vi "SLL DE AI Moving Average V3.0.vi"(8 "error in (no error)":errorcluster, 11 "Input Array":dbl[][](array[numeric])) -> (0 "error out":errorcluster, 3 "Averaged Array":dbl[][](array[numeric]))   [LabVIEW 2013]
uses:
  Controls/SLL DE DAQ Parameters LV2Global Options.ctl
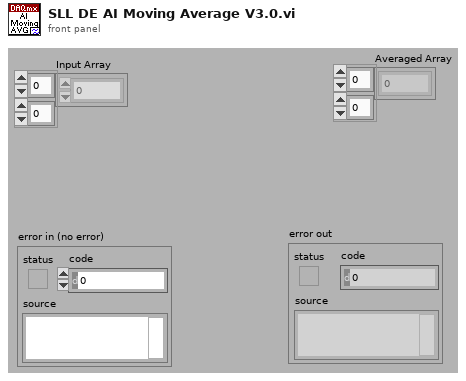
[diagram p1: front panel]
types:
  T1 = typedef "SLL DE DAQ Parameters LV2Global Options.ctl" = enum16{"Read", "Write"}
  T2 = typedef "SLL DE DAQ Engine Parameters.ctl" = cluster{"Enable Engines":cluster{"AI Enable":bool, "AO Enable":bool, "DI Enable":bool, "DO Enable":bool}, "DAQ Control Type":cluster{"Analog Input":enum16{"Finite", "Continuous", "Driver"}, "Analog Output":enum16{"Finite", "Continuous", "Driver"}, "Digital Input":enum16{"Finite", "Continuous", "Driver"}, "Digital Output":enum16{"Finite", "Continuous", "Driver"}}, "DAQ Parameters":cluster{"AI Sampling Rate (Samples/Sec)":dbl, "MvgAVG Window Size (# of Points)":i32, "Enable Filter":bool, "Enable MvgAVG":bool, "Circular Buffer Size (Sec)":dbl, "AO Sampling Rate (Samples/Sec)":dbl, "Graph Update Rate (Samples/Sec)":dbl, "File Logging Rate (Samples/Sec)":i32}, "AO Safe Values":cluster{"Analog Outputs Name":T3, "Analog Outputs Safe Value":dbl}[], "DO Safe Values":cluster{"Digital Outputs Name":T4, "Digital Outputs Safe Value":bool}[], "DO Interconnected Lines":cluster{"First DO Line":string, "Second DO Line":string}[], "AI Channels Unit":cluster{"Channel Name":T5, "Channel Type":T6}[], "Units Information":cluster{"Channel Type":T6, "Unit Text":string, "Maximum":dbl, "Minmum":dbl, "Increments":dbl}[]}
  T3 = typedef "SLL DE List of Analog Outputs.ctl" = enum16{"None"}
  T4 = typedef "SLL DE List of Digital Outputs.ctl" = enum16{"STATION1_START TEST", "STATION1_STOP TEST", "STATION1_LIGHT1", "STATION1_LIGHT2", "STATION1_LIGHT3", "STATION1_SELECT_TEST", "STATION2_START TEST", "STATION2_STOP TEST", "STATION2_LIGHT1", "STATION2_LIGHT2", "STATION2_LIGHT3", "STATION2_SELECT_TEST", "STATION3_START TEST", "STATION3_STOP TEST", "STATION3_LIGHT1", "STATION3_LIGHT2", "STATION3_LIGHT3", "STATION3_SELECT_TEST", "STATION4_START TEST", "STATION4_STOP TEST", "STATION4_LIGHT1", "STATION4_LIGHT2", "STATION4_LIGHT3", "STATION4_SELECT_TEST"}
  T5 = typedef "SLL DE List of Analog Inputs.ctl" = enum16{"None"}
  T6 = typedef "SLL DE List of AI Channel Type.ctl" = enum16{"Pressure", "Flow", "Temperature", "Time Scale", "Voltage", "Current", "Frequency", "Sound", "Speed", "Torque", "Distance", "Channel Type 1", "Channel Type 2", "Channel Type 3"}
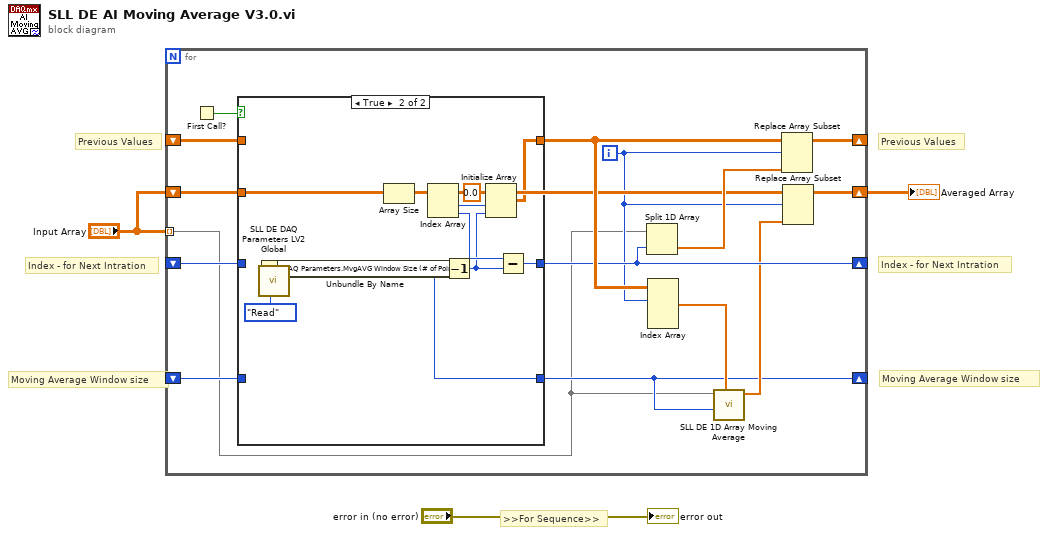
[diagram p0: block diagram]
diagram:
  # ">>For Sequence>>"
  # "Index - for Next Intration"
  # "Index - for Next Intration"
  # "Previous Values"
  # "Previous Values"
  # "Moving Average Window size"
  # "Moving Average Window size"
  n1 = for {
    tunnel: "Input Array" -> [w4] mode=indexing
    shift-right: [w15] -> _
    shift-left: _ -> [w17]
    shift-right: [w12] -> _
    shift-left: _ -> [w11]
    shift-right: [w5] -> _
    shift-left: _ -> [w6]
    shift-right: [w7] -> w2
    shift-left: "Input Array" -> [w10]
    i -> [w9]
    n2 = First Call?() -> (First Call?: T/F=w18:bool)
    n3 = case shown="True" w18 {
      tunnel: [w21 w31] -> w14
      tunnel: w17 -> [w21 _]
      tunnel: w10 -> [_ w30]
      tunnel: [w20 w26] -> w12
      tunnel: w11 -> [w20 _]
      tunnel: [w19 w23] -> w5
      tunnel: w6 -> [w19 _]
      frame False {
      }
      frame True {
        n4 = call "SLL DE DAQ Parameters LV2 Global.vi"("Option"=SLL_DE_DAQ_Parameters_LV2Global_Options."Read") -> ("Global Info"=w25:T2)  [unwired: 9 in, 1 out]
        n5 = Unbundle By Name(w25) -> ("DAQ Parameters.MvgAVG Window Size (# of Points)"=w23:i32)
        n6 = Array Size(array=w30) -> (size(s)=w29:i32[])
        n7 = Index Array(array=w29) -> (element #1=w28:i32, element #2=w27:i32)  [unwired: 2 in]
        n8 = Decrement(x=w23) -> (x-1=w22:i32)
        n9 = Initialize Array(0.0 ("element"), w28, w22) -> (w31:dbl[][])
        n10 = Subtract(x=w27, y=w22) -> (x-y=w26:i32)
      }
    }
    n11 = Split 1D Array(array=w4, index=w12) -> (second subarray=w16:dbl[])  [unwired: 1 out]
    n12 = Index Array(array=w14, index (row) #1=w9) -> (element #1=w13:dbl[])  [unwired: 3 in, 1 out]
    n13 = call "SLL DE 1D Array Moving Average.vi"("Old Points"=w13, "MvgAvg WindowSize"=w5, "Input Array"=w4) -> ("Output Array"=w8:dbl[])  [unwired: 8 in]
    n14 = Replace Array Subset(array=w14, new element=w16, index (row)=w9) -> (w15:dbl[][])  [unwired: 1 in]
    n15 = Replace Array Subset(array=w10, new element=w8, index (row)=w9) -> (w7:dbl[][])  [unwired: 1 in]
  }
  "Averaged Array" <- w2
  "error out" <- "error in (no error)"
